vi "Create Department.vi"(8 "error in (no error)":errorcluster caption="错误输入（无错误）", 11 "Access Factory 输入":refnum<class "Access Factory.lvclass">) -> (0 "error out":errorcluster caption="错误输出", 2 "Abstract Department.lvclass":refnum<class "Abstract Department.lvclass">, 3 "Access Factory 输出":refnum<class "Access Factory.lvclass">)   [LabVIEW 2017, in "Access Factory.lvclass"]
uses:
  Access Factory.lvclass
  Abstract Department/Abstract Department.lvclass
  Access Department/Access Department.lvclass
  Abstract Factory/Abstract Factory.lvclass
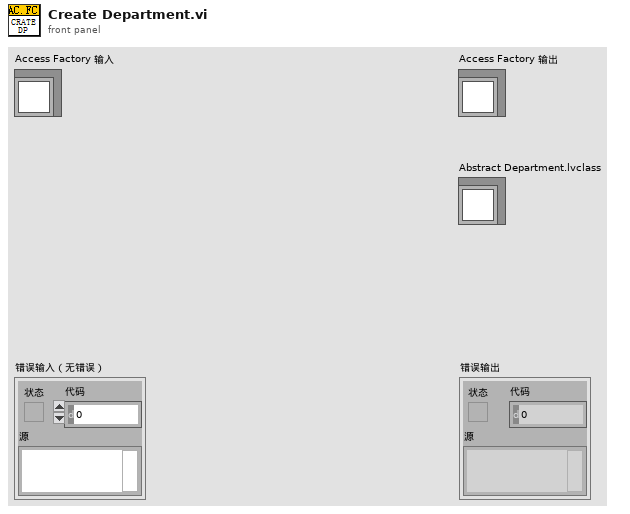
[diagram p1: front panel]
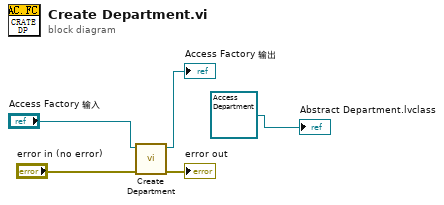
[diagram p0: block diagram]
diagram:
  n1 = call-parent "Create Department.vi"("error in (no error)"="error in (no error)", "Abstract Factory 输入"="Access Factory 输入") -> ("error out"=→"error out":errorcluster, "Abstract Factory 输出"=→"Access Factory 输出":refnum<class "Access Factory.lvclass">)  [unwired: 7 in, 1 out]
  "Abstract Department.lvclass" <- refnum<class "Access Department.lvclass"> refnum ("Access Department.lvclass")
